vi "DrawRGBCurve.vi"(1 "BCurvePos":cluster{i16, i16}[](array[cluster]), 2 "GCurvePos":cluster{i16, i16}[](array[cluster]), 3 "RCurvePos":cluster{i16, i16}[](array[cluster])) -> (0 "Curve in picture":picture)   [LabVIEW 2016]
panel:
  # "Draw the RGB curve seperatly in the picture  by the turn point postion(x,y) array"
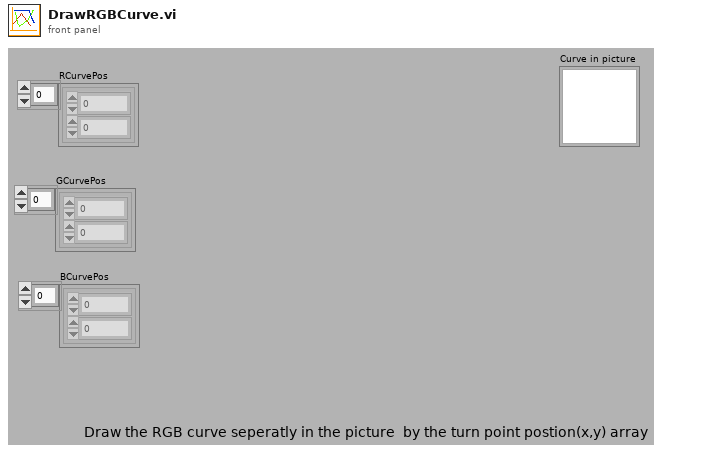
[diagram p1: front panel]
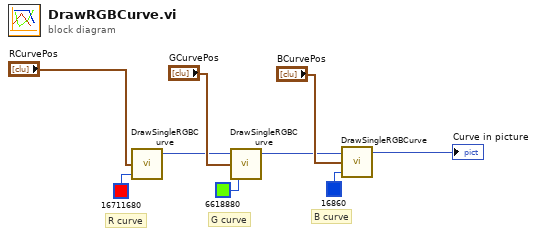
[diagram p0: block diagram]
diagram:
  # "B curve"
  # "R curve"
  # "G curve"
  n1 = call "DrawSingleRGBCurve.vi"("color( default is black)"=u32 16711680 ("color(black)"), "Point Position Cluster Array"="RCurvePos") -> ("new picture"=w2:picture)  [unwired: 2 in, 1 out]
  n2 = call "DrawSingleRGBCurve.vi"("color( default is black)"=u32 6618880 ("color(black)"), "Point Position Cluster Array"="GCurvePos", "picture to be draw curve"=w2) -> ("new picture"=w4:picture)  [unwired: 1 in, 1 out]
  n3 = call "DrawSingleRGBCurve.vi"("color( default is black)"=u32 16860 ("color(black)"), "Point Position Cluster Array"="BCurvePos", "picture to be draw curve"=w4) -> ("new picture"=→"Curve in picture":picture)  [unwired: 1 in, 1 out]
